vi "test_read-nmea-data2.vi"() -> ()   [LabVIEW 2019] (continued)
\t\n15:12:04.58\tF9P\t$GAGSV,2,1,08,02,08,297,10,04,66,118,28,09,32,193,31,11,71,358,32,7*71\n\t\n15:12:04.60\tF9P\t$GAGSV,2,2,08,12,40,102,35,19,26,045,22,25,09,249,,36,26,308,18,7*76\n\t\n15:12:04.62\tF9P\t$GAGSV,2,1,08,02,08,297,,04,66,118,,09,32,193,35,11,71,358,,2*7A\n\t\n15:12:04.64\tF9P\t$GAGSV,2,2,08,12,40,102,,19,26,045,,25,09,249,,36,26,308,,2*7C\n\t\n15:12:04.66\tF9P\t$GBGSV,1,1,03,11,50,132,33,14,87,127,29,33,60,219,29,1*42\n\t\n15:12:04.68\tF9P\t$GBGSV,1,1,03,11,50,132,,14,87,127,34,33,60,219,,3*47\n\t\n15:12:04.70\tF9P\t$GNGLL,3723.53162,N,12656.92763,E,061206.00,A,A*7D\n\t\n15:12:04.72\tF9P\t\t\n15:12:04.74\tF9P\t\t\n15:12:04.76\tF9P\t\t\n15:12:04.78\tF9P\t\t\n15:12:04.80\tF9P\t\t\n15:12:04.82\tF9P\t\t\n15:12:04.84\tF9P\t\t\n15:12:04.86\tF9P\t\t\n15:12:04.88\tF9P\t\t\n15:12:04.90\tF9P\t\t\n15:12:04.92\tF9P\t\t\n15:12:04.94\tF9P\t\t\n15:12:04.96\tF9P\t\t\n15:12:04.98\tF9P\t\t\n15:12:05.00\tF9P\t\t\n15:12:05.02\tF9P\t\t\n15:12:05.04\tF9P\t\t\n15:12:05.06\tF9P\t\t\n15:12:05.08\tF9P\t\t\n15:12:05.10\tF9P\t\t\n15:12:05.12\tF9P\t\t\n15:12:05.14\tF9P\t\t\n15:12:05.16\tF9P\t\t\n15:12:05.18\tF9P\t\t\n15:12:05.20\tF9P\t\t\n15:12:05.22\tF9P\t\t\n15:12:05.24\tF9P\t$GNRMC,061207.00,A,3723.53205,N,12656.92820,E,2.342,48.34,250720,,,A,V*35\n\t\n15:12:05.26\tF9P\t$GNVTG,48.34,T,,M,2.342,N,4.338,K,A*13\n\t\n15:12:05.28\tF9P\t$GNGGA,061207.00,3723.53205,N,12656.92820,E,1,12,0.83,35.2,M,18.5,M,,*73\n\t\n15:12:05.30\tF9P\t$GNGSA,A,3,12,06,19,05,17,09,04,02,,,,,1.56,0.83,1.32,1*09\n\t\n15:12:05.32\tF9P\t$GNGSA,A,3,85,70,71,84,,,,,,,,,1.56,0.83,1.32,2*0B\n\t\n15:12:05.34\tF9P\t$GNGSA,A,3,36,19,11,04,09,12,,,,,,,1.56,0.83,1.32,3*09\n\t\n15:12:05.36\tF9P\t$GNGSA,A,3,14,11,33,,,,,,,,,,1.56,0.83,1.32,4*08\n\t\n15:12:05.38\tF9P\t$GPGSV,3,1,09,02,55,319,38,04,18,043,25,05,37,247,37,06,64,049,27,1*68\n\t\n15:12:05.40\tF9P\t$GPGSV,3,2,09,09,45,074,29,12,23,276,23,17,33,153,35,19,53,157,33,1*66\n\t\n15:12:05.42\tF9P\t$GPGSV,3,3,09,25,12,307,09,1*54\n\t\n15:12:05.44\tF9P\t$GPGSV,3,1,09,02,55,319,,04,18,043,19,05,37,247,24,06,64,049,25,6*6B\n\t\n15:12:05.46\tF9P\t$GPGSV,3,2,09,09,45,074,24,12,23,276,20,17,33,153,22,19,53,157,,6*69\n\t\n15:12:05.48\tF9P\t$GPGSV,3,3,09,25,12,307,,6*5A\n\t\n15:12:05.50\tF9P\t$GLGSV,2,1,08,69,12,031,,70,71,039,33,71,52,205,44,72,04,209,24,1*7C\n\t\n15:12:05.52\tF9P\t$GLGSV,2,2,08,77,01,326,,84,20,122,09,85,70,067,38,86,37,330,,1*7A\n\t\n15:12:05.54\tF9P\t$GLGSV,2,1,08,69,12,031,,70,71,039,,71,52,205,25,72,04,209,,3*7F\n\t\n15:12:05.56\tF9P\t$GLGSV,2,2,08,77,01,326,,84,20,122,12,85,70,067,27,86,37,330,,3*7C\n\t\n15:12:05.58\tF9P\t$GAGSV,2,1,08,02,08,297,11,04,66,118,28,09,32,193,30,11,71,358,28,7*7A\n\t\n15:12:05.60\tF9P\t$GAGSV,2,2,08,12,40,102,27,19,26,045,20,25,09,249,,36,26,308,19,7*76\n\t\n15:12:05.62\tF9P\t$GAGSV,2,1,08,02,08,297,,04,66,118,,09,32,193,34,11,71,358,,2*7B\n\t\n15:12:05.64\tF9P\t$GAGSV,2,2,08,12,40,102,,19,26,045,,25,09,249,,36,26,308,,2*7C\n\t\n15:12:05.66\tF9P\t$GBGSV,1,1,03,11,50,132,25,14,87,127,32,33,60,219,34,1*43\n\t\n15:12:05.68\tF9P\t$GBGSV,1,1,03,11,50,132,,14,87,127,34,33,60,219,,3*47\n\t\n15:12:05.70\tF9P\t$GNGLL,3723.53205,N,12656.92820,E,061207.00,A,A*76\n\t\n15:12:05.72\tF9P\t\t\n15:12:05.74\tF9P\t\t\n15:12:05.76\tF9P\t\t\n15:12:05.78\tF9P\t\t\n15:12:05.80\tF9P\t\t\n15:12:05.82\tF9P\t\t\n15:12:05.84\tF9P\t\t\n15:12:05.86\tF9P\t\t\n15:12:05.88\tF9P\t\t\n15:12:05.90\tF9P\t\t\n15:12:05.92\tF9P\t\t\n15:12:05.94\tF9P\t\t\n15:12:05.96\tF9P\t\t\n15:12:05.98\tF9P\t\t\n15:12:06.00\tF9P\t\t\n15:12:06.02\tF9P\t\t\n15:12:06.04\tF9P\t\t\n15:12:06.06\tF9P\t\t\n15:12:06.08\tF9P\t\t\n15:12:06.10\tF9P\t\t\n15:12:06.12\tF9P\t\t\n15:12:06.14\tF9P\t\t\n15:12:06.16\tF9P\t\t\n15:12:06.18\tF9P\t\t\n15:12:06.20\tF9P\t\t\n15:12:06.22\tF9P\t\t\n15:12:06.24\tF9P\t$GNRMC,061208.00,A,3723.53243,N,12656.92840,E,1.414,37.81,250720,,,A,V*3F\n\t\n15:12:06.26\tF9P\t$GNVTG,37.81,T,,M,1.414,N,2.619,K,A*12\n\t\n15:12:06.28\tF9P\t$GNGGA,061208.00,3723.53243,N,12656.92840,E,1,12,0.85,35.8,M,18.5,M,,*74\n\t\n15:12:06.30\tF9P\t$GNGSA,A,3,12,06,19,05,17,09,04,02,,,,,1.58,0.85,1.33,1*00\n\t\n15:12:06.32\tF9P\t$GNGSA,A,3,85,70,71,84,,,,,,,,,1.58,0.85,1.33,2*02\n\t\n15:12:06.34\tF9P\t$GNGSA,A,3,36,19,11,04,09,12,,,,,,,1.58,0.85,1.33,3*00\n\t\n15:12:06.36\tF9P\t$GNGSA,A,3,14,11,33,,,,,,,,,,1.58,0.85,1.33,4*01\n\t\n15:12:06.38\tF9P\t$GPGSV,3,1,09,02,55,319,41,04,18,043,24,05,37,247,26,06,64,049,34,1*65\n\t\n15:12:06.40\tF9P\t$GPGSV,3,2,09,09,45,074,33,12,23,276,24,17,33,154,35,19,53,157,30,1*6E\n\t\n15:12:06.42\tF9P\t$GPGSV,3,3,09,25,12,307,09,1*54\n\t\n15:12:06.44\tF9P\t$GPGSV,3,1,09,02,55,319,,04,18,043,16,05,37,247,22,06,64,049,31,6*67\n\t\n15:12:06.46\tF9P\t$GPGSV,3,2,09,09,45,074,31,12,23,276,16,17,33,154,26,19,53,157,,6*6B\n\t\n15:12:06.48\tF9P\t$GPGSV,3,3,09,25,12,307,,6*5A\n\t\n15:12:06.50\tF9P\t$GLGSV,2,1,08,69,12,031,,70,71,039,28,71,52,205,42,72,04,209,23,1*77\n\t\n15:12:06.52\tF9P\t$GLGSV,2,2,08,77,01,326,,84,20,122,09,85,70,067,36,86,37,330,,1*74\n\t\n15:12:06.54\tF9P\t$GLGSV,2,1,08,69,12,031,,70,71,039,,71,52,205,30,72,04,209,,3*7B\n\t\n15:12:06.56\tF9P\t$GLGSV,2,2,08,77,01,326,,84,20,122,13,85,70,067,26,86,37,330,,3*7C\n\t\n15:12:06.58\tF9P\t$GAGSV,2,1,08,02,08,297,10,04,66,118,29,09,32,193,32,11,71,358,26,7*76\n\t\n15:12:06.60\tF9P\t$GAGSV,2,2,08,12,40,102,28,19,26,045,21,25,09,249,,36,26,308,21,7*73\n\t\n15:12:06.62\tF9P\t$GAGSV,2,1,08,02,08,297,,04,66,118,,09,32,193,34,11,71,358,,2*7B\n\t\n15:12:06.64\tF9P\t$GAGSV,2,2,08,12,40,102,,19,26,045,,25,09,249,,36,26,308,,2*7C\n\t\n15:12:06.66\tF9P\t$GBGSV,1,1,03,11,50,132,32,14,87,127,32,33,60,219,36,1*47\n\t\n15:12:06.68\tF9P\t$GBGSV,1,1,03,11,50,132,,14,87,127,33,33,60,219,,3*40\n\t\n15:12:06.70\tF9P\t$GNGLL,3723.53243,N,12656.92840,E,061208.00,A,A*7D\n\t\n15:12:06.72\tF9P\t\t\n15:12:06.74\tF9P\t\t\n15:12:06.76\tF9P\t\t\n15:12:06.78\tF9P\t\t\n15:12:06.80\tF9P\t\t\n15:12:06.82\tF9P\t\t\n15:12:06.84\tF9P\t\t\n15:12:06.86\tF9P\t\t\n15:12:06.88\tF9P\t\t\n15:12:06.90\tF9P\t\t\n15:12:06.92\tF9P\t\t\n15:12:06.94\tF9P\t\t\n15:12:06.96\tF9P\t\t\n15:12:06.98\tF9P\t\t\n15:12:07.00\tF9P\t\t\n15:12:07.02\tF9P\t\t\n15:12:07.04\tF9P\t\t\n15:12:07.06\tF9P\t\t\n15:12:07.08\tF9P\t\t\n15:12:07.10\tF9P\t\t\n15:12:07.12\tF9P\t\t\n15:12:07.14\tF9P\t\t\n15:12:07.16\tF9P\t\t\n15:12:07.18\tF9P\t\t\n15:12:07.20\tF9P\t\t\n15:12:07.22\tF9P\t\t\n15:12:07.24\tF9P\t$GNRMC,061209.00,A,3723.53297,N,12656.92866,E,2.110,33.29,250720,,,A,V*37\n\t\n15:12:07.26\tF9P\t$GNVTG,33.29,T,,M,2.110,N,3.907,K,A*17\n\t\n15:12:07.28\tF9P\t$GNGGA,061209.00,3723.53297,N,12656.92866,E,1,12,0.83,34.7,M,18.5,M,,*70\n\t\n15:12:07.30\tF9P\t$GNGSA,A,3,12,06,19,05,17,09,04,02,,,,,1.56,0.83,1.32,1*09\n\t\n15:12:07.32\tF9P\t$GNGSA,A,3,85,70,71,84,,,,,,,,,1.56,0.83,1.32,2*0B\n\t\n15:12:07.34\tF9P\t$GNGSA,A,3,36,19,11,04,09,12,,,,,,,1.56,0.83,1.32,3*09\n\t\n15:12:07.36\tF9P\t$GNGSA,A,3,14,11,33,,,,,,,,,,1.56,0.83,1.32,4*08\n\t\n15:12:07.38\tF9P\t$GPGSV,3,1,09,02,55,319,32,04,18,043,23,05,37,247,39,06,64,049,32,1*6E\n\t\n15:12:07.40\tF9P\t$GPGSV,3,2,09,09,45,074,32,12,23,276,30,17,33,154,35,19,53,157,30,1*6A\n\t\n15:12:07.42\tF9P\t$GPGSV,3,3,09,25,12,307,09,1*54\n\t\n15:12:07.44\tF9P\t$GPGSV,3,1,09,02,55,319,,04,18,043,15,05,37,247,25,06,64,049,27,6*64\n\t\n15:12:07.46\tF9P\t$GPGSV,3,2,09,09,45,074,26,12,23,276,16,17,33,154,25,19,53,157,,6*6E\n\t\n15:12:07.48\tF9P\t$GPGSV,3,3,09,25,12,307,,6*5A\n\t\n15:12:07.50\tF9P\t$GLGSV,2,1,08,69,12,031,,70,71,039,28,71,52,205,35,72,04,209,22,1*76\n\t\n15:12:07.52\tF9P\t$GLGSV,2,2,08,77,01,326,,84,20,122,08,85,70,067,33,86,37,330,,1*70\n\t\n15:12:07.54\tF9P\t$GLGSV,2,1,08,69,12,031,,70,71,039,,71,52,205,29,72,04,209,,3*73\n\t\n15:12:07.56\tF9P\t$GLGSV,2,2,08,77,01,326,,84,20,122,11,85,70,067,24,86,37,330,,3*7C\n\t\n15:12:07.58\tF9P\t$GAGSV,2,1,08,02,08,297,10,04,66,118,26,09,32,193,31,11,71,358,25,7*79\n\t\n15:12:07.60\tF9P\t$GAGSV,2,2,08,12,40,102,27,19,26,045,21,25,09,249,,36,26,308,21,7*7C\n\t\n15:12:07.62\tF9P\t$GAGSV,2,1,08,02,08,297,,04,66,118,,09,32,193,,11,71,358,,2*7C\n\t\n15:12:07.64\tF9P\t$GAGSV,2,2,08,12,40,102,,19,26,045,,25,09,249,,36,26,308,,2*7C\n\t\n15:12:07.66\tF9P\t$GBGSV,1,1,03,11,50,132,28,14,87,127,27,33,60,219,34,1*4A\n\t\n15:12:07.68\tF9P\t$GBGSV,1,1,03,11,50,132,26,14,87,127,28,33,60,219,,3*4E\n\t\n15:12:07.70\tF9P\t$GNGLL,3723.53297,N,12656.92866,E,061209.00,A,A*71\n\t\n15:12:07.72\tF9P\t\t\n15:12:07.74\tF9P\t\t\n15:12:07.76\tF9P\t\t\n15:12:07.78\tF9P\t\t\n15:12:07.80\tF9P\t\t\n15:12:07.82\tF9P\t\t\n15:12:07.84\tF9P\t\t\n15:12:07.86\tF9P\t\t\n15:12:07.88\tF9P\t\t\n15:12:07.90\tF9P\t\t\n15:12:07.92\tF9P\t\t\n15:12:07.94\tF9P\t\t\n15:12:07.96\tF9P\t\t\n15:12:07.98\tF9P\t\t\n15:12:08.00\tF9P\t\t\n15:12:08.02\tF9P\t\t\n15:12:08.04\tF9P\t\t\n15:12:08.06\tF9P\t\t\n15:12:08.08\tF9P\t\t\n15:12:08.10\tF9P\t\t\n15:12:08.12\tF9P\t\t\n15:12:08.14\tF9P\t\t\n15:12:08.16\tF9P\t\t\n15:12:08.18\tF9P\t\t\n15:12:08.20\tF9P\t\t\n15:12:08.22\tF9P\t\t\n15:12:08.24\tF9P\t$GNRMC,061210.00,A,3723.53336,N,12656.92923,E,1.997,40.99,250720,,,A,V*3E\n\t\n15:12:08.26\tF9P\t$GNVTG,40.99,T,,M,1.997,N,3.699,K,A*14\n\t\n15:12:08.28\tF9P\t$GNGGA,061210.00,3723.53336,N,12656.92923,E,1,12,0.72,35.4,M,18.5,M,,*7E\n\t\n15:12:08.30\tF9P\t$GNGSA,A,3,12,06,19,05,17,09,04,02,,,,,1.33,0.72,1.12,1*06\n\t\n15:12:08.32\tF9P\t$GNGSA,A,3,85,70,71,84,,,,,,,,,1.33,0.72,1.12,2*04\n\t\n15:12:08.34\tF9P\t$GNGSA,A,3,36,19,11,04,09,12,,,,,,,1.33,0.72,1.12,3*06\n\t\n15:12:08.36\tF9P\t$GNGSA,A,3,14,11,33,,,,,,,,,,1.33,0.72,1.12,4*07\n\t\n15:12:08.38\tF9P\t$GPGSV,3,1,09,02,55,319,29,04,18,043,22,05,37,247,31,06,64,049,36,1*69\n\t\n15:12:08.40\tF9P\t$GPGSV,3,2,09,09,45,074,34,12,23,276,30,17,33,154,31,19,52,157,29,1*61\n\t\n15:12:08.42\tF9P\t$GPGSV,3,3,09,25,12,307,12,1*5E\n\t\n15:12:08.44\tF9P\t$GPGSV,3,1,09,02,55,319,,04,18,043,15,05,37,247,26,06,64,049,31,6*60\n\t\n15:12:08.46\tF9P\t$GPGSV,3,2,09,09,45,074,30,12,23,276,15,17,33,154,25,19,52,157,,6*6B\n\t\n15:12:08.48\tF9P\t$GPGSV,3,3,09,25,12,307,,6*5A\n\t\n15:12:08.50\tF9P\t$GLGSV,2,1,08,69,12,031,,70,71,039,29,71,52,205,37,72,04,209,25,1*72\n\t\n15:12:08.52\tF9P\t$GLGSV,2,2,08,77,01,326,,84,20,122,10,85,70,067,38,86,37,330,,1*72\n\t\n15:12:08.54\tF9P\t$GLGSV,2,1,08,69,12,031,,70,71,039,,71,52,205,23,72,04,209,,3*79\n\t\n15:12:08.56\tF9P\t$GLGSV,2,2,08,77,01,326,,84,20,122,14,85,70,067,24,86,37,330,,3*79\n\t\n15:12:08.58\tF9P\t$GAGSV,2,1,08,02,08,297,11,04,66,118,28,09,32,193,35,11,71,358,31,7*77\n\t\n15:12:08.60\tF9P\t$GAGSV,2,2,08,12,40,102,27,19,26,045,22,25,09,249,,36,26,308,19,7*74\n\t\n15:12:08.62\tF9P\t$GAGSV,2,1,08,02,08,297,,04,66,118,,09,32,193,,11,71,358,,2*7C\n\t\n15:12:08.64\tF9P\t$GAGSV,2,2,08,12,40,102,,19,26,045,,25,09,249,,36,26,308,,2*7C\n\t\n15:12:08.66\tF9P\t$GBGSV,1,1,04,11,50,132,29,14,87,127,26,28,,,34,33,60,219,34,1*40\n\t\n15:12:08.68\tF9P\t$GBGSV,1,1,03,11,50,132,32,14,87,127,,33,60,219,,3*41\n\t\n15:12:08.70\tF9P\t$GNGLL,3723.53336,N,12656.92923,E,061210.00,A,A*73\n\t\n15:12:08.72\tF9P\t\t\n15:12:08.74\tF9P\t\t\n15:12:08.76\tF9P\t\t\n15:12:08.78\tF9P\t\t\n15:12:08.80\tF9P\t\t\n15:12:08.82\tF9P\t\t\n15:12:08.84\tF9P\t\t\n15:12:08.86\tF9P\t\t\n15:12:08.88\tF9P\t\t\n15:12:08.90\tF9P\t\t\n15:12:08.92\tF9P\t\t\n15:12:08.94\tF9P\t\t\n15:12:08.96\tF9P\t\t\n15:12:08.98\tF9P\t\t\n15:12:09.00\tF9P\t\t\n15:12:09.02\tF9P\t\t\n15:12:09.04\tF9P\t\t\n15:12:09.06\tF9P\t\t\n15:12:09.08\tF9P\t\t\n15:12:09.10\tF9P\t\t\n15:12:09.12\tF9P\t\t\n15:12:09.14\tF9P\t\t\n15:12:09.16\tF9P\t\t\n15:12:09.18\tF9P\t\t\n15:12:09.20\tF9P\t\t\n15:12:09.22\tF9P\t\t\n15:12:09.24\tF9P\t$GNRMC,061211.00,A,3723.53366,N,12656.92988,E,1.948,52.66,250720,,,A,V*3A\n\t\n15:12:09.26\tF9P\t$GNVTG,52.66,T,,M,1.948,N,3.608,K,A*1D\n\t\n15:12:09.28\tF9P\t$GNGGA,061211.00,3723.53366,N,12656.92988,E,1,12,0.73,36.7,M,18.5,M,,*7A\n\t\n15:12:09.30\tF9P\t$GNGSA,A,3,12,06,19,05,17,09,04,02,,,,,1.35,0.73,1.14,1*07\n\t\n15:12:09.32\tF9P\t$GNGSA,A,3,85,70,71,84,,,,,,,,,1.35,0.73,1.14,2*05\n\t\n15:12:09.34\tF9P\t$GNGSA,A,3,36,19,11,04,09,12,,,,,,,1.35,0.73,1.14,3*07\n\t\n15:12:09.36\tF9P\t$GNGSA,A,3,14,11,33,,,,,,,,,,1.35,0.73,1.14,4*06\n\t\n15:12:09.38\tF9P\t$GPGSV,3,1,09,02,55,319,22,04,18,043,21,05,37,247,25,06,64,049,28,1*6B\n\t\n15:12:09.40\tF9P\t$GPGSV,3,2,09,09,45,074,34,12,23,276,26,17,33,154,36,19,52,157,29,1*61\n\t\n15:12:09.42\tF9P\t$GPGSV,3,3,09,25,12,307,14,1*58\n\t\n15:12:09.44\tF9P\t$GPGSV,3,1,09,02,55,319,,04,18,043,14,05,37,247,27,06,64,049,25,6*65\n\t\n15:12:09.46\tF9P\t$GPGSV,3,2,09,09,45,074,29,12,23,276,17,17,33,154,23,19,52,157,,6*67\n\t\n15:12:09.48\tF9P\t$GPGSV,3,3,09,25,12,307,,6*5A\n\t\n15:12:09.50\tF9P\t$GLGSV,2,1,08,69,12,031,,70,71,039,33,71,52,205,40,72,04,209,30,1*7D\n\t\n15:12:09.52\tF9P\t$GLGSV,2,2,08,77,01,326,,84,20,122,09,85,70,067,40,86,37,330,,1*75\n\t\n15:12:09.54\tF9P\t$GLGSV,2,1,08,69,12,031,,70,71,039,,71,52,205,22,72,04,209,,3*78\n\t\n15:12:09.56\tF9P\t$GLGSV,2,2,08,77,01,326,,84,20,122,10,85,70,067,23,86,37,330,,3*7A\n\t\n15:12:09.58\tF9P\t$GAGSV,2,1,08,02,08,297,11,04,66,117,28,09,32,193,37,11,71,358,35,7*7E\n\t\n15:12:09.60\tF9P\t$GAGSV,2,2,08,12,40,102,33,19,26,045,21,25,09,249,,36,26,308,20,7*78\n\t\n15:12:09.62\tF9P\t$GAGSV,2,1,08,02,08,297,,04,66,117,,09,32,193,,11,71,358,,2*73\n\t\n15:12:09.64\tF9P\t$GAGSV,2,2,08,12,40,102,,19,26,045,,25,09,249,,36,26,308,,2*7C\n\t\n15:12:09.66\tF9P\t$GBGSV,1,1,04,11,50,132,30,14,87,127,32,28,,,33,33,60,219,34,1*4A\n\t\n15:12:09.68\tF9P\t$GBGSV,1,1,03,11,50,132,28,14,87,127,31,33,60,219,,3*48\n\t\n15:12:09.70\tF9P\t$GNGLL,3723.53366,N,12656.92988,E,061211.00,A,A*76\n\t\n15:12:09.72\tF9P\t\t\n15:12:09.74\tF9P\t\t\n15:12:09.76\tF9P\t\t\n15:12:09.78\tF9P\t\t\n15:12:09.80\tF9P\t\t\n15:12:09.82\tF9P\t\t\n15:12:09.84\tF9P\t\t\n15:12:09.86\tF9P\t\t\n15:12:09.88\tF9P\t\t\n15:12:09.90\tF9P\t\t\n15:12:09.92\tF9P\t\t\n15:12:09.94\tF9P\t\t\n15:12:09.96\tF9P\t\t\n15:12:09.98\tF9P\t\t\n15:12:10.00\tF9P\t\t\n15:12:10.02\tF9P\t\t\n15:12:10.04\tF9P\t\t\n15:12:10.06\tF9P\t\t\n15:12:10.08\tF9P\t\t\n15:12:10.10\tF9P\t\t\n15:12:10.12\tF9P\t\t\n15:12:10.14\tF9P\t\t\n15:12:10.16\tF9P\t\t\n15:12:10.18\tF9P\t\t\n15:12:10.20\tF9P\t\t\n15:12:10.22\tF9P\t\t\n15:12:10.24\tF9P\t$GNRMC,061212.00,A,3723.53377,N,12656.93064,E,2.084,70.99,250720,,,A,V*39\n\t\n15:12:10.26\tF9P\t$GNVTG,70.99,T,,M,2.084,N,3.860,K,A*17\n\t\n15:12:10.28\tF9P\t$GNGGA,061212.00,3723.53377,N,12656.93064,E,1,12,0.83,38.4,M,18.5,M,,*71\n\t\n15:12:10.30\tF9P\t$GNGSA,A,3,12,06,19,05,17,09,04,02,,,,,1.56,0.83,1.32,1*09\n\t\n15:12:10.32\tF9P\t$GNGSA,A,3,85,70,71,84,,,,,,,,,1.56,0.83,1.32,2*0B\n\t\n15:12:10.34\tF9P\t$GNGSA,A,3,36,19,11,04,09,12,,,,,,,1.56,0.83,1.32,3*09\n\t\n15:12:10.36\tF9P\t$GNGSA,A,3,14,11,33,,,,,,,,,,1.56,0.83,1.32,4*08\n\t\n15:12:10.38\tF9P\t$GPGSV,3,1,09,02,55,319,29,04,18,043,20,05,37,247,43,06,64,049,29,1*60\n\t\n15:12:10.40\tF9P\t$GPGSV,3,2,09,09,45,074,29,12,23,276,37,17,33,154,34,19,52,157,33,1*64\n\t\n15:12:10.42\tF9P\t$GPGSV,3,3,09,25,12,307,14,1*58\n\t\n15:12:10.44\tF9P\t$GPGSV,3,1,09,02,55,319,,04,18,043,,05,37,247,26,06,64,049,25,6*61\n\t\n15:12:10.46\tF9P\t$GPGSV,3,2,09,09,45,074,28,12,23,276,18,17,33,154,23,19,52,157,,6*69\n\t\n15:12:10.48\tF9P\t$GPGSV,3,3,09,25,12,307,,6*5A\n\t\n15:12:10.50\tF9P\t$GLGSV,2,1,08,69,12,031,,70,71,039,35,71,52,205,40,72,04,209,24,1*7E\n\t\n15:12:10.52\tF9P\t$GLGSV,2,2,08,77,01,326,,84,20,122,09,85,70,067,31,86,37,330,,1*73\n\t\n15:12:10.54\tF9P\t$GLGSV,2,1,08,69,12,031,,70,71,039,,71,52,205,24,72,04,209,,3*7E\n\t\n15:12:10.56\tF9P\t$GLGSV,2,2,08,77,01,326,,84,20,122,07,85,70,067,22,86,37,330,,3*7D\n\t\n15:12:10.58\tF9P\t$GAGSV,2,1,08,02,08,297,08,04,66,117,29,09,32,193,33,11,71,358,32,7*74\n\t\n15:12:10.60\tF9P\t$GAGSV,2,2,08,12,40,102,27,19,26,045,19,25,09,249,,36,26,308,21,7*77\n\t\n15:12:10.62\tF9P\t$GAGSV,2,1,08,02,08,297,,04,66,117,,09,32,193,,11,71,358,,2*73\n\t\n15:12:10.64\tF9P\t$GAGSV,2,2,08,12,40,102,,19,26,045,,25,09,249,,36,26,308,,2*7C\n\t\n15:12:10.66\tF9P\t$GBGSV,1,1,04,11,50,132,26,14,87,127,31,28,,,22,33,60,219,34,1*4E\n\t\n15:12:10.68\tF9P\t$GBGSV,1,1,03,11,50,132,27,14,87,127,26,33,60,219,,3*41\n\t\n15:12:10.70\tF9P\t$GNGLL,3723.53377,N,12656.93064,E,061212.00,A,A*7F\n\t\n15:12:10.72\tF9P\t\t\n15:12:10.74\tF9P\t\t\n15:12:10.76\tF9P\t\t\n15:12:10.78\tF9P\t\t\n15:12:10.80\tF9P\t\t\n15:12:10.82\tF9P\t\t\n15:12:10.84\tF9P\t\t\n15:12:10.86\tF9P\t\t\n15:12:10.88\tF9P\t\t\n15:12:10.90\tF9P\t\t\n15:12:10.93\tF9P\t\t\n15:12:10.95\tF9P\t\t\n15:12:10.97\tF9P\t\t\n15:12:10.99\tF9P\t\t\n15:12:11.01\tF9P\t\t\n15:12:11.03\tF9P\t\t\n15:12:11.05\tF9P\t\t\n15:12:11.07\tF9P\t\t\n15:12:11.09\tF9P\t\t\n15:12:11.11\tF9P\t\t\n15:12:11.13\tF9P\t\t\n15:12:11.15\tF9P\t\t\n15:12:11.17\tF9P\t\t\n15:12:11.19\tF9P\t\t\n15:12:11.21\tF9P\t\t\n15:12:11.23\tF9P\t\t\n15:12:11.25\tF9P\t$GNRMC,061213.00,A,3723.53433,N,12656.93119,E,2.545,52.43,250720,,,A,V*3B\n\t\n15:12:11.27\tF9P\t$GNVTG,52.43,T,,M,2.545,N,4.714,K,A*13\n\t\n15:12:11.29\tF9P\t$GNGGA,061213.00,3723.53433,N,12656.93119,E,1,12,0.72,38.3,M,18.5,M,,*75\n\t\n15:12:11.31\tF9P\t$GNGSA,A,3,12,06,19,05,17,09,04,02,,,,,1.33,0.72,1.12,1*06\n\t\n15:12:11.33\tF9P\t$GNGSA,A,3,85,70,71,84,,,,,,,,,1.33,0.72,1.12,2*04\n\t\n15:12:11.35\tF9P\t$GNGSA,A,3,36,19,11,04,09,12,,,,,,,1.33,0.72,1.12,3*06\n\t\n15:12:11.37\tF9P\t$GNGSA,A,3,14,11,33,,,,,,,,,,1.33,0.72,1.12,4*07\n\t\n15:12:11.39\tF9P\t$GPGSV,3,1,09,02,55,319,22,04,18,043,19,05,37,247,34,06,64,049,33,1*6A\n\t\n15:12:11.41\tF9P\t$GPGSV,3,2,09,09,45,074,27,12,23,276,30,17,33,154,37,19,52,157,38,1*65\n\t\n15:12:11.43\tF9P\t$GPGSV,3,3,09,25,12,307,14,1*58\n\t\n15:12:11.45\tF9P\t$GPGSV,3,1,09,02,55,319,,04,18,043,,05,37,247,24,06,64,049,26,6*60\n\t\n15:12:11.47\tF9P\t$GPGSV,3,2,09,09,45,074,20,12,23,276,18,17,33,154,23,19,52,157,,6*61\n\t\n15:12:11.49\tF9P\t$GPGSV,3,3,09,25,12,307,,6*5A\n\t\n15:12:11.51\tF9P\t$GLGSV,2,1,08,69,12,031,,70,71,039,28,71,52,205,43,72,04,209,23,1*76\n\t\n15:12:11.53\tF9P\t$GLGSV,2,2,08,77,01,326,,84,20,122,10,85,70,067,38,86,37,330,,1*72\n\t\n15:12:11.55\tF9P\t$GLGSV,2,1,08,69,12,031,,70,71,039,,71,52,205,22,72,04,209,,3*78\n\t\n15:12:11.57\tF9P\t$GLGSV,2,2,08,77,01,326,,84,20,122,07,85,70,067,20,86,37,330,,3*7F\n\t\n15:12:11.59\tF9P\t$GAGSV,2,1,08,02,08,297,07,04,66,117,28,09,32,193,38,11,71,358,28,7*7A\n\t\n15:12:11.61\tF9P\t$GAGSV,2,2,08,12,40,102,27,19,26,045,16,25,09,249,,36,26,308,20,7*79\n\t\n15:12:11.63\tF9P\t$GAGSV,2,1,08,02,08,297,,04,66,117,,09,32,193,,11,71,358,,2*73\n\t\n15:12:11.65\tF9P\t$GAGSV,2,2,08,12,40,102,,19,26,045,,25,09,249,,36,26,308,,2*7C\n\t\n15:12:11.67\tF9P\t$GBGSV,1,1,04,11,50,132,32,14,87,127,31,28,,,23,33,60,219,30,1*4E\n\t\n15:12:11.69\tF9P\t$GBGSV,1,1,03,11,50,132,27,14,87,127,31,33,60,219,,3*47\n\t\n15:12:11.71\tF9P\t$GNGLL,3723.53433,N,12656.93119,E,061213.00,A,A*72\n\t\n15:12:11.73\tF9P\t\t\n15:12:11.75\tF9P\t\t\n15:12:11.77\tF9P\t\t\n15:12:11.79\tF9P\t\t\n15:12:11.81\tF9P\t\t\n15:12:11.83\tF9P\t\t\n15:12:11.85\tF9P\t\t\n15:12:11.87\tF9P\t\t\n15:12:11.89\tF9P\t\t\n15:12:11.91\tF9P\t\t\n15:12:11.93\tF9P\t\t\n15:12:11.95\tF9P\t\t\n15:12:11.97\tF9P\t\t\n15:12:11.99\tF9P\t\t\n15:12:12.01\tF9P\t\t\n15:12:12.03\tF9P\t\t\n15:12:12.05\tF9P\t\t\n15:12:12.07\tF9P\t\t\n15:12:12.09\tF9P\t\t\n15:12:12.11\tF9P\t\t\n15:12:12.13\tF9P\t\t\n15:12:12.15\tF9P\t\t\n15:12:12.17\tF9P\t\t\n15:12:12.19\tF9P\t\t\n15:12:12.21\tF9P\t\t\n15:12:12.23\tF9P\t$GNRMC,061214.00,A,3723.53484,N,12656.93169,E,1.713,50.38,250720\t\n15:12:12.25\tF9P\t,,,A,V*3B\n\t\n15:12:12.27\tF9P\t$GNVTG,50.38,T,,M,1.713,N,3.173,K,A*1F\n\t\n15:12:12.29\tF9P\t$GNGGA,061214.00,3723.53484,N,12656.93169,E,1,12,0.72,38.3,M,18.5,M,,*79\n\t\n15:12:12.31\tF9P\t$GNGSA,A,3,12,06,19,05,17,09,04,02,,,,,1.33,0.72,1.12,1*06\n\t\n15:12:12.33\tF9P\t$GNGSA,A,3,85,70,71,84,,,,,,,,,1.33,0.72,1.12,2*04\n\t\n15:12:12.35\tF9P\t$GNGSA,A,3,36,19,11,04,09,12,,,,,,,1.33,0.72,1.12,3*06\n\t\n15:12:12.37\tF9P\t$GNGSA,A,3,14,11,33,,,,,,,,,,1.33,0.72,1.12,4*07\n\t\n15:12:12.39\tF9P\t$GPGSV,3,1,09,02,55,319,21,04,18,043,20,05,37,247,34,06,64,049,33,1*63\n\t\n15:12:12.41\tF9P\t$GPGSV,3,2,09,09,45,074,28,12,23,276,30,17,33,154,30,19,52,157,31,1*64\n\t\n15:12:12.43\tF9P\t$GPGSV,3,3,09,25,12,307,14,1*58\n\t\n15:12:12.45\tF9P\t$GPGSV,3,1,09,02,55,319,,04,
